vi "CalibrateStartPosition.vi"(10 "Start Position [mm]":dbl[](array[numeric]), 11 ".NET Refnum In":refnum<k24>) -> (2 "Final Position [mm]":dbl[](array[numeric]))   [LabVIEW 2016]
uses:
  C:/Users/Aerotech/Documents/BNLStaveAssembly-blueprint/Bin/Aerotech.A3200.dll
  BNLStaveAssembly-blueprint/Bin/Aerotech.A3200.dll
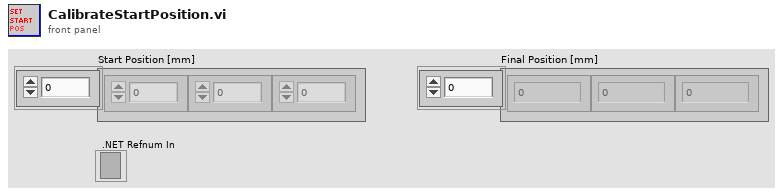
[diagram p1: front panel]
types:
  T1 = cluster{"Final X":dbl, "Final Y":dbl, "Final Z":dbl}
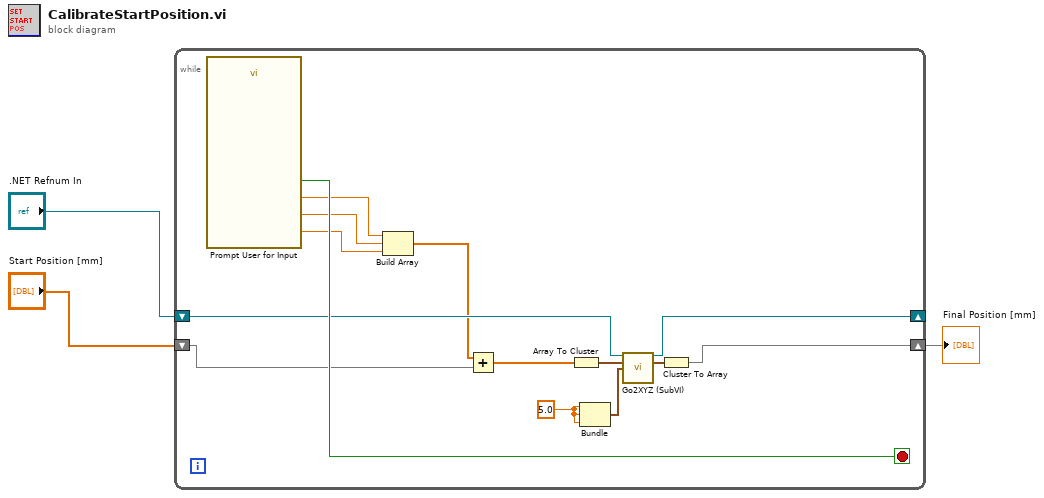
[diagram p0: block diagram]
diagram:
  n1 = while {
    shift-right: [w15] -> w1
    shift-left: "Start Position [mm]" -> [w6]
    shift-right: [w13] -> _
    shift-left: ".NET Refnum In" -> [w14]
    stop <- w17 stop-if-true
    w11 = 5.0
    n2 = call "Prompt User for Input"() -> ("Adjust z [mm]"=w8:dbl, "Adjust y [mm]"=w9:dbl, "Adjust x [mm]"=w10:dbl, "Accept"=w17:bool)  [unwired: 14 in, 2 out]
    n3 = Build Array(w10, w9, w8) -> (w5:dbl[])
    n4 = Add(x=w5, y=w6) -> (x+y=w7:dbl[])
    n5 = Array To Cluster(array=w7) -> (cluster=w4:cluster{"[0]":dbl, "[1]":dbl, "[2]":dbl})
    n6 = Bundle(w11, w11, w11) -> (w12:cluster{dbl, dbl, dbl})  [unwired: 1 in]
    n7 = call "Go2XYZ (SubVI).vi"(".NET Refnum in"=w14, "Go to Coordinates"=w4, "Axis Speeds"=w12) -> (".NET Refnum out"=w13:refnum<k24>, "Final Position"=w16:T1)  [unwired: 8 in, 3 out]
    n8 = Cluster To Array(cluster=w16) -> (array=w15:dbl[])
  }
  "Final Position [mm]" <- w1
